vi "Read commandName.vi"(8 "error in (no error)":errorcluster, 11 "StopImageCapture in":refnum<class "StopImageCapture.lvclass">) -> (0 "error out":errorcluster, 2 "CommandValue":T1, 3 "StopImageCapture out":refnum<class "StopImageCapture.lvclass">)   [LabVIEW 2016, in "Commands.lvlib" / "StopImageCapture.lvclass"]
uses:
  StopImageCapture.lvclass
  Typedefs/CommandValue.ctl
  Typedefs/EXATypedefs.lvlib
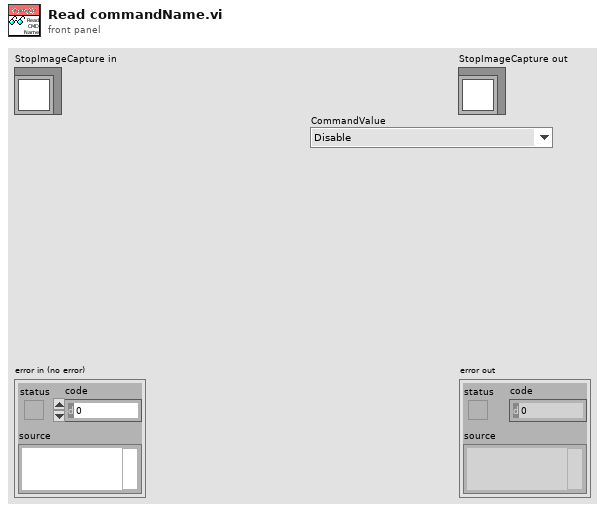
[diagram p1: front panel]
types:
  T1 = typedef "EXATypedefs.lvlib/CommandValue.ctl" = enum16{"Disable", "Enable", "Exit", "GoToStandby", "OnHeartbeat", "OnIncomingMessagingError", "OnInterrupt", "Start"}
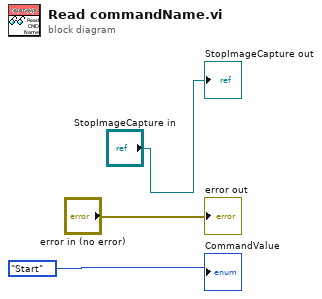
[diagram p0: block diagram]
diagram:
  "error out" <- "error in (no error)"
  "StopImageCapture out" <- "StopImageCapture in"
  "CommandValue" <- CommandValue."Start" ("CommandValue")
